vi "MODE_GET_FORMAT.vi"(11 "DATA":u8[](array[numeric])) -> (3 "MOTOR_PARAM":T1={"DRIVER_MODE"=enum."VOLTAGE", "MOTOR_Type_42"=enum."Unknown", "MICROSTEPPING"=enum."1", "WORK_CURRENT"=enum."0.1A", "STOP_CURRENT"=enum."25%"})   [LabVIEW 2021, in "SMSD.lvclass"]
uses:
  SMSD.lvclass
  Ctl/MOTOR_PARAM.ctl
  Ctl/DRIVER_MODE.ctl
  Ctl/MOTOR_Type_42.ctl
  Ctl/MICROSTEPPING.ctl
  Ctl/WORK_CURRENT.ctl
  Ctl/STOP_CURRENT.ctl
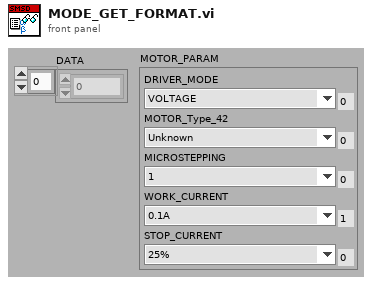
[diagram p1: front panel]
types:
  T1 = typedef "SMSD.lvclass/MOTOR_PARAM.ctl" = cluster{"DRIVER_MODE":T2, "MOTOR_Type_42":T3, "MICROSTEPPING":T4, "WORK_CURRENT":T5, "STOP_CURRENT":T6}
  T2 = typedef "SMSD.lvclass/DRIVER_MODE.ctl" = enum16{"VOLTAGE", "CURRENT"}
  T3 = typedef "SMSD.lvclass/MOTOR_Type_42.ctl" = enum16{"Unknown", "FL42STH33-1334 1.8 deg", "FL42STH33-1334 0.9 deg", "FL42STH38-1206 0.9 deg", "FL42STH38-1684 1.8 deg", "FL42STH38-1684 0.9 deg", "FL42STH47-1206 1.8 deg", "FL42STH47-1684 1.8 deg", "FL42STH47-1684 0.9 deg", "FL42STH60-1206 1.8 deg", "FL42STH60-1206 0.9 deg", "FL57ST41-1564 1.8 deg", "FL57ST76-1006 1.8 deg", "FL57ST76-1506 1.8 deg", "FL57STH41-1006 1.8 deg", "FL57STH41-1006 0.9 deg", "FL57STH41-2804 1.8 deg", "FL57STH41-2804 0.9 deg", "FL57STH51-1006 1.8 deg", "FL57STH51-2804 1.8 deg", "FL57STH51-2804 0.9 deg", "FL57STH56-1006 1.8 deg", "FL57STH56-2006 1.8 deg", "FL57STH56-2804 1.8 deg", "FL57STH76-1006 1.8 deg", "FL57STH76-2804 1.8 deg", "FL57STH76-2804 0.9 deg", "FL60STH65-2008 1.8 deg parallel", "FL60STH65-2008 1.8 deg serial", "FL60STH86-2008 1.8 deg parallel", "FL60STH86-2008 1.8 deg serial", "FL86STH65-2808 1.8 deg parallel", "FL86STH65-2808 1.8 deg serial", "FL86STH80-4208 1.8 deg parallel", "FL86STH80-4208 1.8 deg serial", "FL86STH118-4208 1.8 deg parallel", "FL86STH118-4208 1.8 deg serial", "FL86STH156-4208 1.8 deg parallel", "FL86STH156-4208 1.8 deg serial", "ДШ3934-0,3А", "ДШ2851-0,7А", "ДШ4248-1,7A", "ДШ5776-3,0А", "ДШ57112-3,0А", "ДШ8665-3,0А", "ДШ8682-4,5А"}
  T4 = typedef "SMSD.lvclass/MICROSTEPPING.ctl" = enum16{"1", "1/2", "1/4", "1/8", "1/16", "1/32", "1/64", "1/128"}
  T5 = typedef "SMSD.lvclass/WORK_CURRENT.ctl" = enum16{"0.0A", "0.1A", "0.2A", "0.3A", "0.4A", "0.5A", "0.6A", "0.7A", "0.8A", "0.9A", "1.0A", "1.1A", "1.2A", "1.3A", "1.4A", "1.5A", "1.6A", "1.7A", "1.8A", "1.9A", "2.0A", "2.1A", "2.2A", "2.3A", "2.4A", "2.5A", "2.6A", "2.7A", "2.8A", "2.9A", "3.0A", "3.1A", "3.2A", "3.3A", "3.4A", "3.5A", "3.6A", "3.7A", "3.8A", "3.9A", "4.0A", "4.1A", "4.2A"}
  T6 = typedef "SMSD.lvclass/STOP_CURRENT.ctl" = enum16{"25%", "50%", "75%", "100%"}
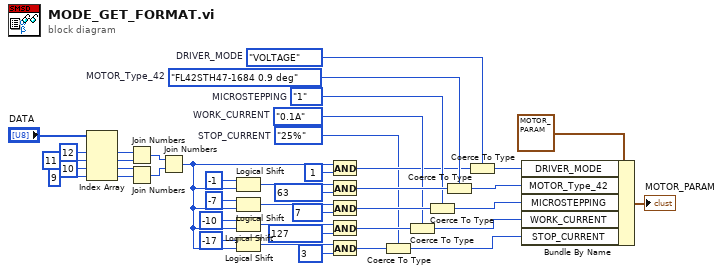
[diagram p0: block diagram]
diagram:
  w8 = STOP_CURRENT."25%"  # STOP_CURRENT
  w14 = DRIVER_MODE."VOLTAGE"  # DRIVER_MODE
  w34 = WORK_CURRENT."0.1A"  # WORK_CURRENT
  w35 = MICROSTEPPING."1"  # MICROSTEPPING
  w36 = MOTOR_Type_42."FL42STH47-1684 0.9 deg"  # MOTOR_Type_42
  n1 = Index Array(array="DATA", index #1=12 ("index"), index #2=11 ("index"), index #3=10 ("index"), index #4=9 ("index")) -> (element #1=w23:u8, element #2=w22:u8, element #3=w21:u8, element #4=w20:u8)
  n2 = Join Numbers(hi=w23, lo=w22) -> ((hi.lo)=w19:u16)
  n3 = Join Numbers(hi=w21, lo=w20) -> ((hi.lo)=w18:u16)
  n4 = Join Numbers(hi=w19, lo=w18) -> ((hi.lo)=w10:u32)
  n5 = Logical Shift(y=i16 -1, x=w10) -> (x << y=w37:u32)
  n6 = Logical Shift(y=i16 -7, x=w10) -> (x << y=w38:u32)
  n7 = Logical Shift(y=i16 -10, x=w10) -> (x << y=w39:u32)
  n8 = Logical Shift(y=i16 -17, x=w10) -> (x << y=w11:u32)
  n9 = And(x=w10, y=u32 1) -> (x .and. y?=w15:u32)
  n10 = And(x=w37, y=u32 63) -> (x .and. y?=w42:u32)
  n11 = And(x=w38, y=u32 7) -> (x .and. y?=w41:u32)
  n12 = And(x=w39, y=u32 127) -> (x .and. y?=w40:u32)
  n13 = And(x=w11, y=u32 3) -> (x .and. y?=w9:u32)
  n14 = Coerce To Type(0:w9, 1:w8) -> (2:w2:T6)
  n15 = Coerce To Type(0:w40, 1:w34) -> (2:w3:T5)
  n16 = Coerce To Type(0:w41, 1:w35) -> (2:w4:T4)
  n17 = Coerce To Type(0:w42, 1:w36) -> (2:w5:T3)
  n18 = Coerce To Type(0:w15, 1:w14) -> (2:w6:T2)
  n19 = Bundle By Name(cluster=T1 {"DRIVER_MODE"=enum."VOLTAGE", "MOTOR_Type_42"=enum."Unknown", "MICROSTEPPING"=enum."1", "WORK_CURRENT"=enum."0.1A", "STOP_CURRENT"=enum."25%"} ("MOTOR_PARAM"), "DRIVER_MODE"=w6, "MOTOR_Type_42"=w5, "MICROSTEPPING"=w4, "WORK_CURRENT"=w3, "STOP_CURRENT"=w2) -> (→"MOTOR_PARAM":T1)
